vi "Read Output.vi"(8 "error in (no error)":errorcluster, 11 "CallVIStep in":refnum<class "CallVIStep.lvclass">) -> (0 "error out":errorcluster, 2 "Output":T1[](array[typedef]), 3 "CallVIStep out":refnum<class "CallVIStep.lvclass">)   [LabVIEW 2015, in "CallVIStep.lvclass"]
uses:
  CallVIStep.lvclass
  Step/STEP_OUTPUT.ctl
  Step/OUTPUT_DATA_TYPE.ctl
  OutputUI/OUTPUT_CHECK_TYPE.ctl
  Step/OUTPUT_VALUE_TYPE.ctl
  Step.lvclass
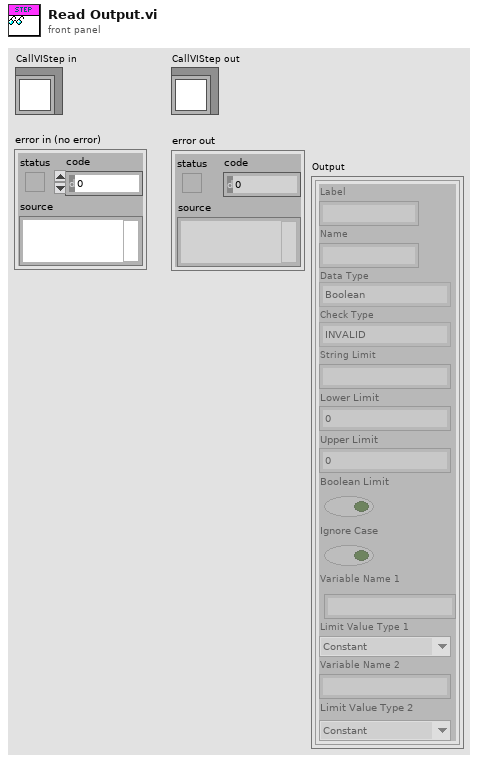
[diagram p1: front panel]
types:
  T1 = typedef "Step.lvclass/STEP_OUTPUT.ctl" = cluster{"Label":string, "Name":string, "Data Type":T2, "Check Type":T3, "String Limit":string, "Lower Limit":dbl, "Upper Limit":dbl, "Boolean Limit":bool, "Ignore Case":bool, "Variable Name 1":string, "Limit Value Type 1":T4, "Variable Name 2":string, "Limit Value Type 2":T4}
  T2 = typedef "Step.lvclass/OUTPUT_DATA_TYPE.ctl" = enum16{"Boolean", "String", "Numeric", "Other"}
  T3 = typedef "Step.lvclass/OUTPUT_CHECK_TYPE.ctl" = enum16{"INVALID", "DO_NOT_CHECK", "RECORD", "VARIABLE", "EQUAL", "NOT_EQUAL", "STR_CONTAINS", "STR_START_WITH", "STR_END_WITH", "STR_REGEX_MATCH", "NUM_GT", "NUM_LT", "NUM_GE", "NUM_LE", "NUM_RANGE", "NUM_RANGE_BDY"}
  T4 = typedef "Step.lvclass/OUTPUT_VALUE_TYPE.ctl" = enum16{"Constant", "Variable"}
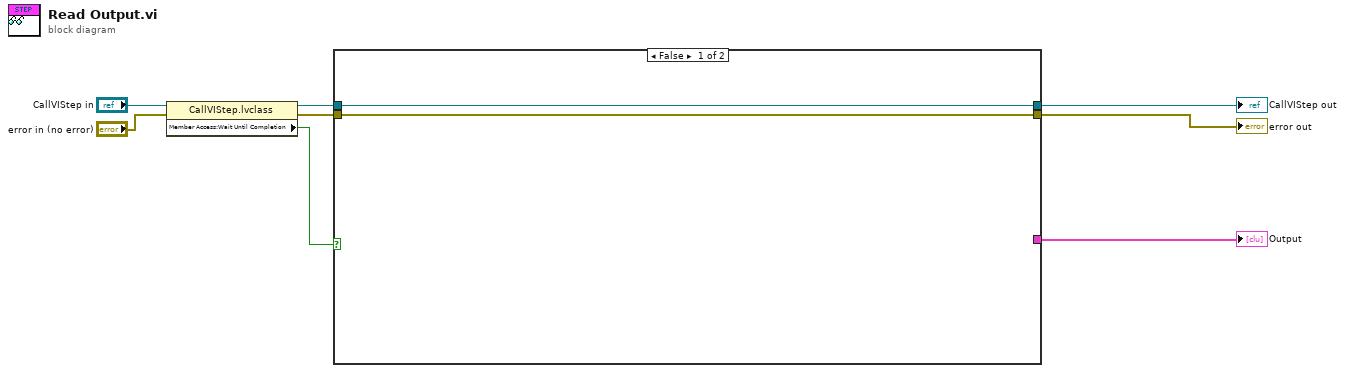
[diagram p0: block diagram]
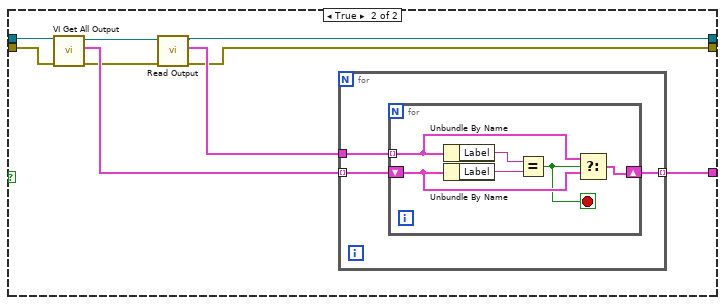
[diagram p2: hidden frame]
diagram:
  n1 = property class="CallVIStep.lvclass"(reference="CallVIStep in", error in="error in (no error)") -> (reference out=w4:refnum<class "CallVIStep.lvclass">, error out=w2:errorcluster, "Member Access:Wait Until Completion"=w1:bool)
  n2 = case shown="False" w1 {
    tunnel: [_ w18] -> w8
    tunnel: [w10 w14] -> w7
    tunnel: [w9 w13] -> w6
    tunnel: w4 -> [w10 w12]
    tunnel: w2 -> [w9 w11]
    frame False {
    }
    frame True {
      n3 = call-dynamic "VI Get All Output.vi"("error in (no error)"=w11, "CallVIStep in"=w12) -> ("error out"=w16:errorcluster, "Output"=w19:T1[], "CallVIStep out"=w17:refnum<class "CallVIStep.lvclass">)  [unwired: 7 in]
      n4 = call-parent "Read Output.vi"("error in (no error)"=w16, "Step in"=w17) -> ("error out"=w13:errorcluster, "Output"=w15:T1[], "Step out"=w14:refnum<class "CallVIStep.lvclass">)  [unwired: 7 in]
      n5 = for {
        tunnel: w19 -> [w21] mode=indexing
        tunnel: w15 -> [w22]
        tunnel: [w20] -> w18 mode=indexing
        n6 = for {
          tunnel: w22 -> [w26] mode=indexing
          shift-right: [w24] -> w20
          shift-left: w21 -> [w25]
          stop <- w23 stop-if-true
          n7 = Unbundle By Name(w26) -> ("Label"=w27:string)
          n8 = Unbundle By Name(w25) -> ("Label"=w28:string)
          n9 = Equal?(x=w27, y=w28) -> (x = y?=w23:bool)
          n10 = Select(t=w26, s=w23, f=w25) -> (s? t:f=w24:T1)
        }
      }
    }
  }
  "error out" <- w6
  "CallVIStep out" <- w7
  "Output" <- w8
